vi "test.Launcher.vi"() -> ()   [LabVIEW 2017, in "TimerEngine.lvlib"]
uses:
  TimerEngine.lvlib
  TimerEngine.lvclass
panel:
  in  "rename timer1":bool
  out "ready?":bool
  in  "enable 2":bool=TRUE
  in  "enable 1":bool=TRUE
  out "diff 1":dbl
  out "diff 2":dbl
  in  "TimePeroid(ms)":i32=1000
  out "Timer Descriptions":string[](array[string])
  in  "unregister timer1":bool
  in  "unregister timer2":bool
  out "[current time]":timestamp
  out "current time 2":timestamp
  out "Event Time Stamp 2":timestamp
  out "Event Time Stamp":timestamp
  out "current time":timestamp
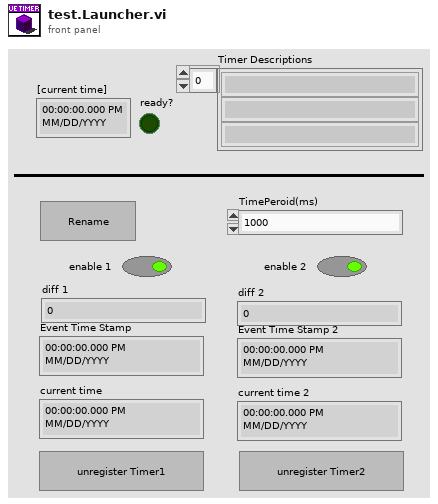
[diagram p1: front panel]
types:
  T1 = typedef "TimerEngine.lvlib/TimerEngine.lvclass/Timer-Userevent.ctl" = refnum<user-event>
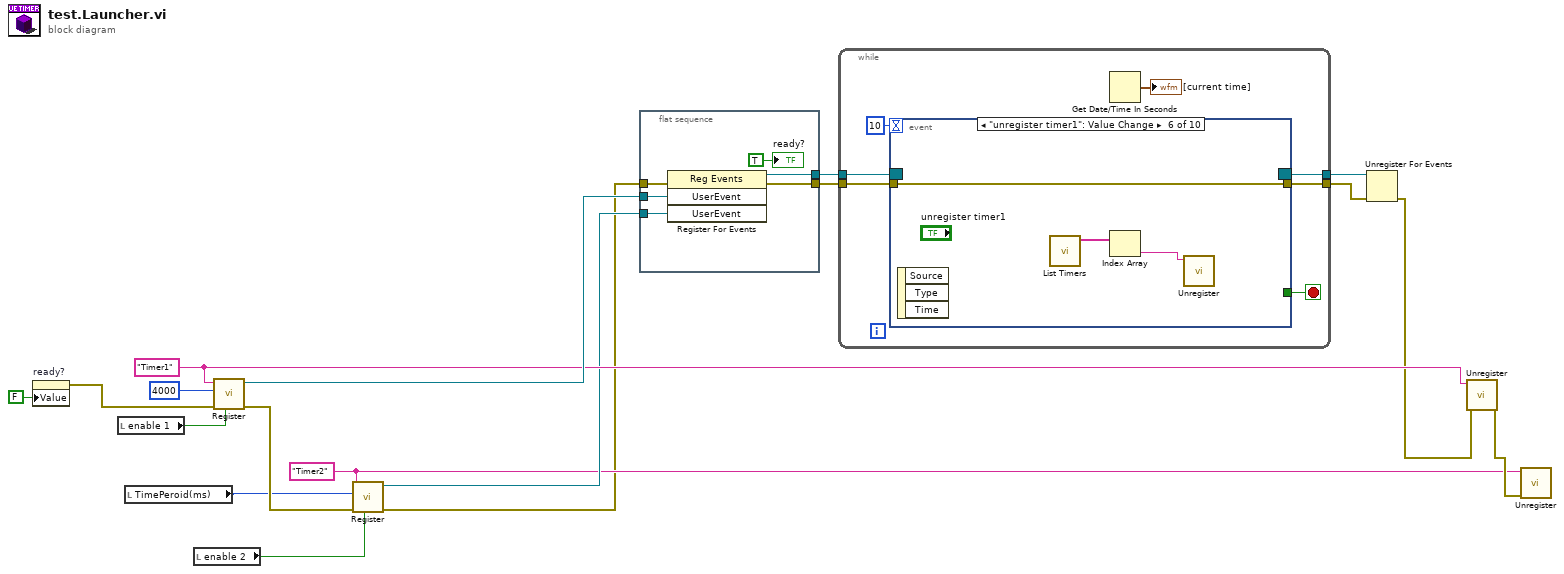
[diagram p0: block diagram]
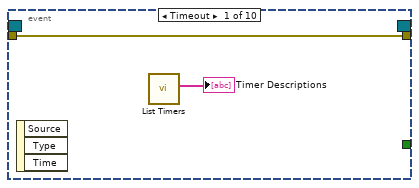
[diagram p2: hidden frame]
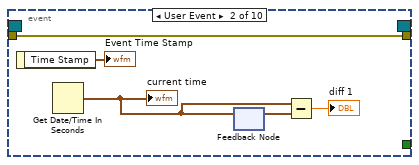
[diagram p3: hidden frame]
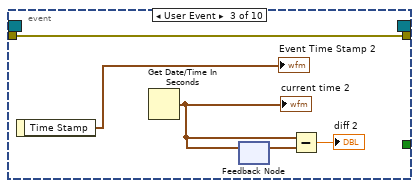
[diagram p4: hidden frame]
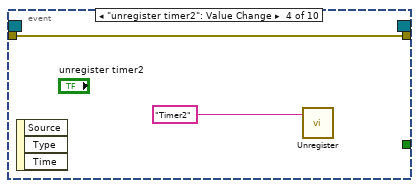
[diagram p5: hidden frame]
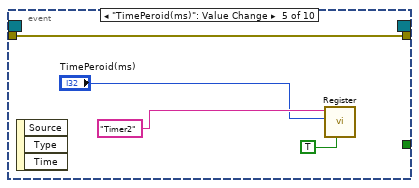
[diagram p6: hidden frame]
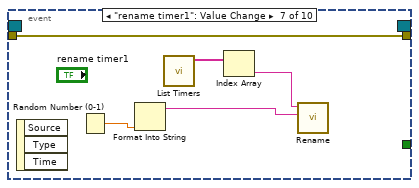
[diagram p7: hidden frame]
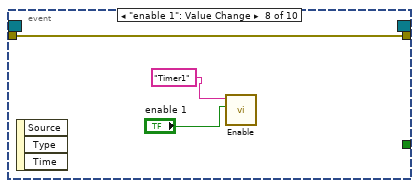
[diagram p8: hidden frame]
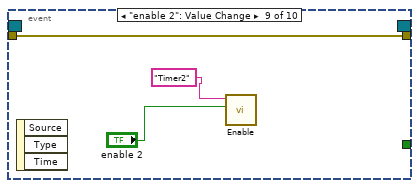
[diagram p9: hidden frame]
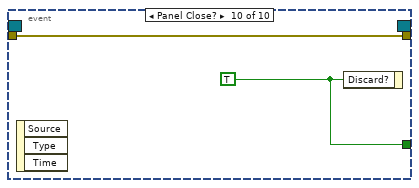
[diagram p10: hidden frame]
diagram:
  w7 = "Timer2" ("Name")
  w12 = "Timer1" ("Name")
  n1 = property on="ready?" class="Bool (strict)"("Value"=FALSE ("ready?")) -> (error out=w1:errorcluster)  [unwired: 2 in, 1 out]
  n2 = local read "enable 1"() -> (w4:bool)
  n3 = local read "TimePeroid(ms)"() -> (w5:i32)
  n4 = local read "enable 2"() -> (w3:bool)
  n5 = call "Register.vi"("Start Imidiatlely?(T)"=w4, "error in (no error)"=w1, "TimePeroid(ms)"=4000, "Name"=w12) -> ("error out"=w9:errorcluster, "UserEvent"=w17:T1)  [unwired: 6 in]
  n6 = call "Register.vi"("Start Imidiatlely?(T)"=w3, "error in (no error)"=w9, "TimePeroid(ms)"=w5, "Name"=w7) -> ("error out"=w6:errorcluster, "UserEvent"=w10:T1)  [unwired: 6 in]
  n7 = flat-sequence {
    tunnel: w17 -> [w24]
    tunnel: [w23] -> w16
    tunnel: [w22] -> w14
    tunnel: w10 -> [w21]
    tunnel: w6 -> [w20]
    frame #0 {
      n8 = register-events(error in=w20, w24, w21) -> (reference out=w23:refnum<event-registration>, error out=w22:errorcluster)  [unwired: 1 in]
      "ready?" <- TRUE ("ready?")
    }
  }
  n9 = while {
    tunnel: w16 -> [w31]
    tunnel: [w29] -> w15
    tunnel: w14 -> [w28]
    tunnel: [w27] -> w13
    stop <- w30 stop-if-true
    n10 = event shown="[5] \"unregister timer1\": Value Change" {
      selector: w31 -> [_ _ _ _ _ _ _ _ _ _]
      dyn-events: [_ _ _ _ _ _ _ _ _ _] -> w29
      timeout: 10 -> [_ _ _ _ _ _ _ _ _ _]
      tunnel: [_ _ _ _ _ _ _ _ _ w65] -> w30
      tunnel: w28 -> [w33 w38 w43 w45 w49 w52 w57 w60 w63 w64]
      tunnel: [w33 w38 w43 w45 w49 w52 w57 w60 w63 w64] -> w27
      event Timeout {
        n11 = event-data() -> ()  [unwired: 1 in, 3 out]
        n12 = call "List Timers.vi"() -> ("Timer Descriptions"=→"Timer Descriptions":string[])  [unwired: 9 in, 2 out]
      }
      event User Event {
        n13 = event-data() -> ("Time Stamp"=→"Event Time Stamp":timestamp)  [unwired: 1 in]
        n14 = Get Date/Time In Seconds() -> (seconds since 1Jan1904=w34:timestamp)
        "current time" <- w34
        n15 = feedback #1() -> (w36:timestamp)  [unwired: 1 in]
        n16 = feedback-in #1(w34) -> ()
        n17 = Subtract(x=w34, y=w36) -> (x-y=→"diff 1":dbl)
      }
      event User Event {
        n18 = event-data() -> ("Time Stamp"=→"Event Time Stamp 2":timestamp)  [unwired: 1 in]
        n19 = Get Date/Time In Seconds() -> (seconds since 1Jan1904=w41:timestamp)
        "current time 2" <- w41
        n20 = feedback-in #2(w41) -> ()
        n21 = feedback #2() -> (w40:timestamp)  [unwired: 1 in]
        n22 = Subtract(x=w41, y=w40) -> (x-y=→"diff 2":dbl)
      }
      event "unregister timer2": Value Change {
        n23 = event-data() -> ()  [unwired: 1 in, 3 out]
        n24 = call "Unregister.vi"("Name"="Timer2") -> ()  [unwired: 10 in, 1 out]
      }
      event "TimePeroid(ms)": Value Change {
        n25 = event-data() -> ()  [unwired: 1 in, 3 out]
        n26 = call "Register.vi"("Start Imidiatlely?(T)"=TRUE ("Start Imidiatlely?(F)"), "TimePeroid(ms)"="TimePeroid(ms)", "Name"="Timer2") -> ()  [unwired: 7 in, 2 out]
      }
      event "unregister timer1": Value Change {
        n27 = event-data() -> ()  [unwired: 1 in, 3 out]
        n28 = call "List Timers.vi"() -> ("Timers"=w51:string[])  [unwired: 9 in, 2 out]
        n29 = Index Array(array=w51) -> (element=w50:string)  [unwired: 1 in]
        n30 = call "Unregister.vi"("Name"=w50) -> ()  [unwired: 10 in, 1 out]
      }
      event "rename timer1": Value Change {
        n31 = event-data() -> ()  [unwired: 1 in, 3 out]
        n32 = Random Number (0-1)() -> (number: 0 to 1=w56:dbl)
        n33 = Format Into String(w56) -> (resulting string=w55:string)  [unwired: 3 in, 1 out]
        n34 = call "List Timers.vi"() -> ("Timers"=w54:string[])  [unwired: 9 in, 2 out]
        n35 = Index Array(array=w54) -> (element=w53:string)  [unwired: 1 in]
        n36 = call "Rename.vi"("New Name"=w55, "Name"=w53) -> ()  [unwired: 9 in, 1 out]
      }
      event "enable 1": Value Change {
        n37 = event-data() -> ()  [unwired: 1 in, 3 out]
        n38 = call "Enable.vi"("Enable?"="enable 1", "Name"="Timer1") -> ()  [unwired: 9 in, 1 out]
      }
      event "enable 2": Value Change {
        n39 = event-data() -> ()  [unwired: 1 in, 3 out]
        n40 = call "Enable.vi"("Enable?"="enable 2", "Name"="Timer2") -> ()  [unwired: 9 in, 1 out]
      }
      event Panel Close? {
        w65 = TRUE ("Discard?")
        n41 = event-data() -> ()  [unwired: 1 in, 3 out]
        n42 = event-data("Discard?"=w65) -> ()  [unwired: 1 in, 1 out]
      }
    }
    n43 = Get Date/Time In Seconds() -> (seconds since 1Jan1904=→"[current time]":timestamp)
  }
  n44 = Unregister For Events(event registration refnum=w15, error in=w13) -> (error out=w11:errorcluster)
  n45 = call "Unregister.vi"("error in (no error)"=w11, "Name"=w12) -> ("error out"=w8:errorcluster)  [unwired: 9 in]
  n46 = call "Unregister.vi"("error in (no error)"=w8, "Name"=w7) -> ()  [unwired: 9 in, 1 out]
